vi "PRUEBA.vi"() -> ()   [LabVIEW 2019]
uses:
  Control 1.ctl
panel:
  in  "Posicion Ascensor":dbl(slide) scale=0.0..100.0
  in  "Selecc. Piso Inicio":enum16{"Piso 1", "Piso 2", "Piso 3", "Piso 4"}(ring)
  in  "Manual-Automatico":bool=TRUE
  in  "Start-Stop":bool
  in  "Cerrar":bool
  in  "Abrir":bool
  out "Bajando":bool
  out "Subiendo":bool
  in  "Piso 4":u16(ring)
  in  "Piso 3":u16(ring)
  in  "Piso 2":u16(ring)
  in  "Piso 1":u16(ring)
  in  "Indicador Cabina":u16(ring)
  out "Bajar 4":bool
  out "Subir 3":bool
  out "Bajar 3":bool
  out "Subir 2":bool
  out "Bajar 2":bool
  out "Subir 1":bool
  out "P02":bool
  out "P04":bool
  out "P01":bool
  out "P03":bool
  in  "Piso 4":bool
  in  "Piso 2":bool
  in  "Piso 3":bool
  in  "Piso 1":bool
  # "0 = Piso 1"
  # "33 = Piso 2"
  # "66 = Piso 3"
  # "100 = Piso 4"
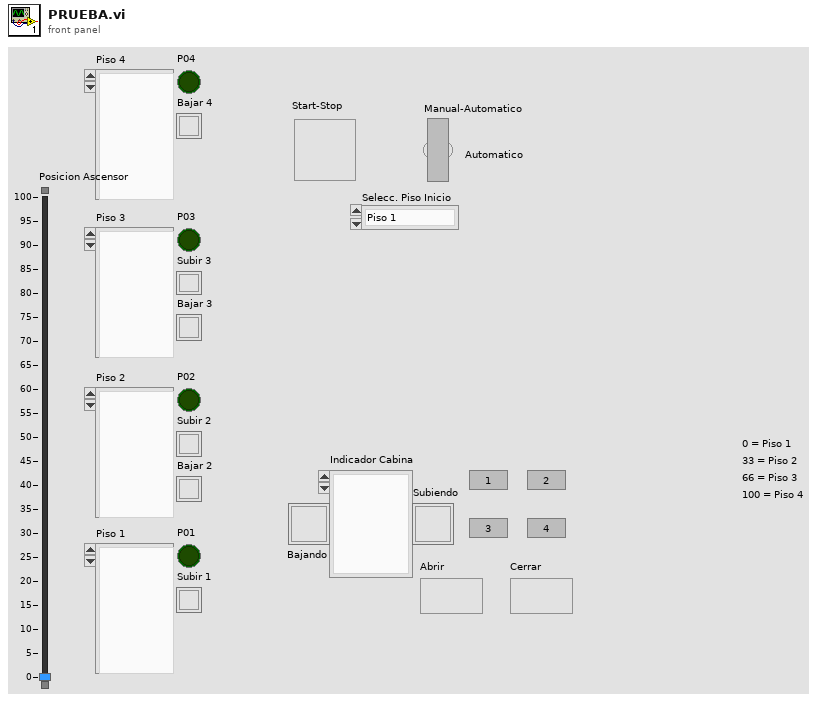
[diagram p1: front panel]
types:
  T1 = typedef "Control 1.ctl" = enum16{"Inicio", "Manual", "Auto", "Piso 1", "Piso 2", "Piso 3", "Piso 4", "Stop", "Start", "Mmto"}
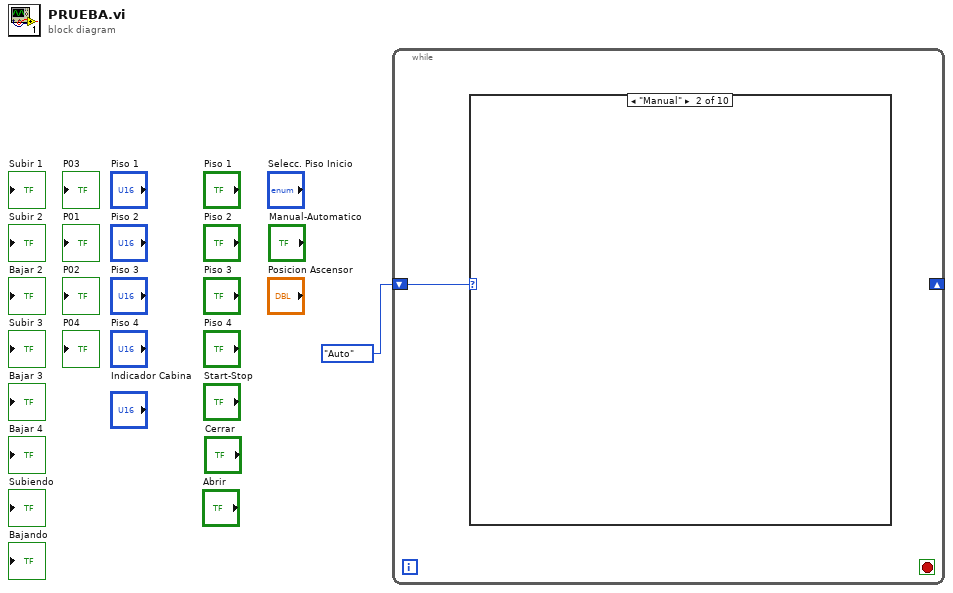
[diagram p0: block diagram]
diagram:
  n1 = while {
    shift-right: _ -> [_]
    shift-left: Control_1."Auto" -> [w2]
    stop <- _ stop-if-true
    n2 = case shown="\"Manual\"" w2 {
      frame "Inicio", Default {
      }
      frame "Manual" {
      }
      frame "Auto" {
      }
      frame "Piso 1" {
      }
      frame "Piso 2" {
      }
      frame "Piso 3" {
      }
      frame "Piso 4" {
      }
      frame "Stop" {
      }
      frame "Start" {
      }
      frame "Mmto" {
      }
    }
  }
